vi "Start Session.vi"(8 "Error In":errorcluster, 11 "MICS Config Cluster":T1 {"flags"."Wake-up Mode" format="%02x"; "flags"."Auto Listen" format="%02x"; "flags"."Auto CCA" format="%02x"; "emergency"."userData" items=["0 - 000", "1 - 001", "2 - 010", "3 - 011", "4 - 100", "5 - 101", "6 - 110", "7 - 111"]; "emergency"."maxBlkPerTxPack" items=["1", "2", "3", "4", "5", "6", "7", "8", "9", "10", "11", "12", "13", "14", "15", "16", "17", "18", "19", "20", "21", "22", "23", "24", "25", "26", "27", "28", "29", "30", "31"]; "emergency"."RxModu" items=["2FSK-FB", "2FSK", "4FSK"]; "emergency"."TxModu" items=["2FSK-FB", "2FSK", "4FSK"]; "emergency"."BlkSize" items=["2", "3", "4", "5", "6", "7", "8", "9", "10", "11", "12", "13", "14", "15", "16", "17", "18", "19", "20", "21", "22", "23", "24", "25", "26", "27", "28", "29", "30", "31"]; "emergency"."chan" items=["0", "1", "2", "3", "4", "5", "6", "7", "8", "9"]; "cal245GTxdBm" items=["-29", "-4", "-2", "0", "2", "4", "6", "8", "10", "12", "14", "16", "18", "20", "22", "24", "26", "27"]; "set245GTxdBm" items=["-29", "-4", "-2", "0", "2", "4", "6", "8", "10", "12", "14", "16", "18", "20", "22", "24", "26", "27"]; "micsRevOnIM" items=["ZL70100", "ZL70101", "ZL70102"]; "CompanyId" format="%02x"; "normal"."userData" items=["0 - 000", "1 - 001", "2 - 010", "3 - 011", "4 - 100", "5 - 101", "6 - 110", "7 - 111"]; "normal"."maxBlkPerTxPack" items=["1", "2", "3", "4", "5", "6", "7", "8", "9", "10", "11", "12", "13", "14", "15", "16", "17", "18", "19", "20", "21", "22", "23", "24", "25", "26", "27", "28", "29", "30", "31"]; "normal"."RxModu" items=["2FSK-FB", "2FSK", "4FSK"]; "normal"."TxModu" items=["2FSK-FB", "2FSK", "4FSK"]; "normal"."BlkSize" items=["2", "3", "4", "5", "6", "7", "8", "9", "10", "11", "12", "13", "14", "15", "16", "17", "18", "19", "20", "21", "22", "23", "24", "25", "26", "27", "28", "29", "30", "31"]; "normal"."chan" items=["0", "1", "2", "3", "4", "5", "6", "7", "8", "9"]; "TransceiverId"."b1" format="%02x"; "TransceiverId"."b2" format="%02x"; "TransceiverId"."b3" format="%02x"}) -> (0 "Error Out":errorcluster, 2 "Base station info":string, 3 "Reference Out":i32)   [LabVIEW 2009]
uses:
  Reference.vi
  MICS Config.ctl
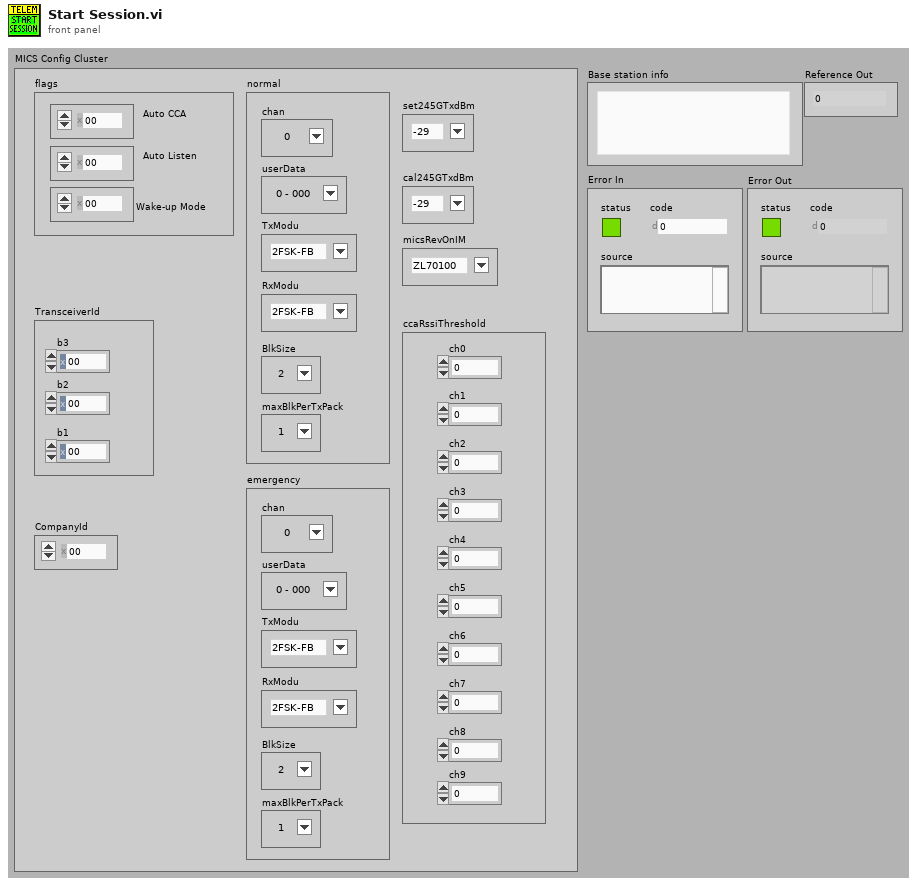
[diagram p1: front panel]
types:
  T1 = typedef "MICS Config.ctl" = cluster{"flags":cluster{"Auto CCA":u8, "Auto Listen":u8, "Wake-up Mode":u8}, "TransceiverId":cluster{"b3":u8, "b2":u8, "b1":u8}, "CompanyId":u8, "normal":cluster{"chan":u8, "userData":u8, "TxModu":u8, "RxModu":u8, "BlkSize":u8, "maxBlkPerTxPack":u8}, "emergency":cluster{"chan":u8, "userData":u8, "TxModu":u8, "RxModu":u8, "BlkSize":u8, "maxBlkPerTxPack":u8}, "set245GTxdBm":i8, "cal245GTxdBm":i8, "micsRevOnIM":u8, "ccaRssiThreshold":cluster{"ch0":u16, "ch1":u16, "ch2":u16, "ch3":u16, "ch4":u16, "ch5":u16, "ch6":u16, "ch7":u16, "ch8":u16, "ch9":u16}}
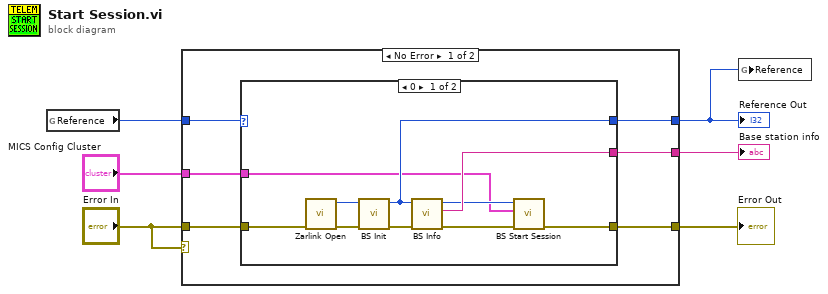
[diagram p0: block diagram]
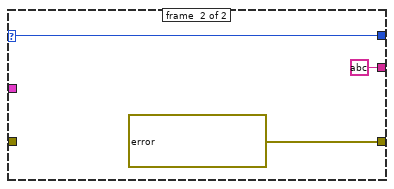
[diagram p2: hidden frame]
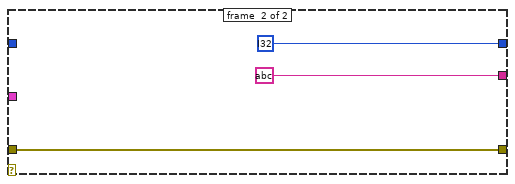
[diagram p3: hidden frame]
diagram:
  n1 = global read "Reference.vi" "Reference"() -> (w1:i32)
  n2 = case shown="No Error" "Error In" {
    tunnel: [w12 string ? ("Result")] -> w6
    tunnel: [w11 i32 ? ("Reference Out")] -> w3
    tunnel: "Error In" -> [w10 w28]
    tunnel: [w9 w28] -> w5
    tunnel: "MICS Config Cluster" -> [w8 _]
    tunnel: w1 -> [w7 _]
    frame #0 {
      n3 = case shown="0" w7 {
        selector: w7 -> [_ w23]
        tunnel: [w22 string ? ("Result")] -> w12
        tunnel: [w21 w23] -> w11
        tunnel: w10 -> [w17 _]
        tunnel: [w15 errorcluster ? ("Error Out")] -> w9
        tunnel: w8 -> [w13 _]
        frame #0 {
          n4 = call <vilib>:"Zarlink Open.vi"("Error In"=w17) -> ("Error Out"=w19:errorcluster, "Reference Out"=w20:i32)  [unwired: 8 in]
          n5 = call <vilib>:"BS Init.vi"("Error In"=w19, "Reference In"=w20) -> ("Error Out"=w18:errorcluster, "Reference Out"=w21:i32)  [unwired: 7 in]
          n6 = call <vilib>:"BS Info.vi"("Error In"=w18, "Reference In"=w21) -> ("Error Out"=w16:errorcluster, "Result"=w22:string, "Reference Out"=w14:i32)  [unwired: 7 in]
          n7 = call <vilib>:"BS Start Session.vi"("Error In"=w16, "MicsConfigCluster"=w13, "Reference In"=w14) -> ("Error Out"=w15:errorcluster)  [unwired: 6 in, 1 out]
        }
        frame #1 {
        }
      }
    }
    frame #1 {
    }
  }
  "Base station info" <- w6
  "Reference Out" <- w3
  "Error Out" <- w5
  n8 = global write "Reference.vi" "Reference"(w3) -> ()
